vi "_Add A New Entry.vi"(4 "Tag Name":string="ChannelDescription", 5 "error in (no error)":errorcluster, 6 "Data":string, 7 "Parent Node":refnum<k20>, 8 "DOM document":refnum<k20>) -> (0 "error out":errorcluster, 2 "Parent Node out":refnum<k20>, 3 "DOM document out":refnum<k20>)   [LabVIEW 2015]
uses:
  <vilib>/xml/Close Reference(Node).vi
  <resource>/objmgr/DOMUserDefRef.rc
  <vilib>/xml/NI_XML.lvlib
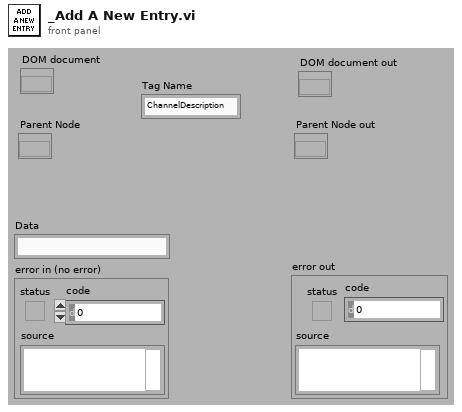
[diagram p1: front panel]
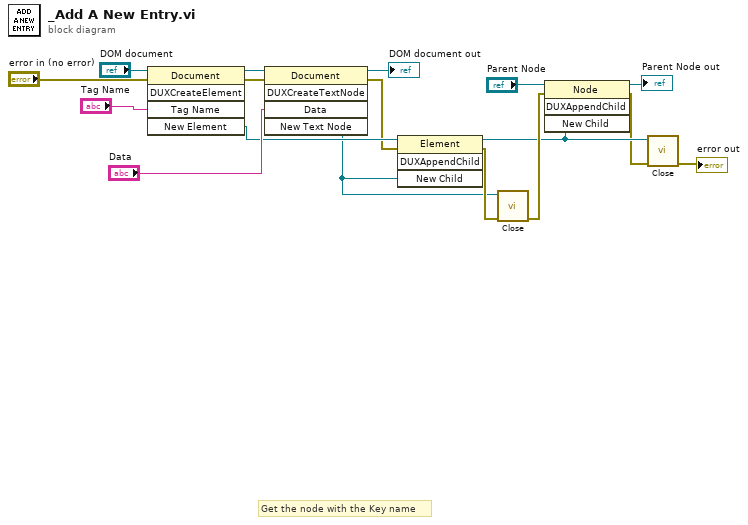
[diagram p0: block diagram]
diagram:
  # "Get the node with the Key name"
  n1 = invoke class="Document" method="DUXCreateElement"(reference="DOM document", error in="error in (no error)", "Tag Name"="Tag Name") -> (reference out=w15:refnum<k20>, error out=w14:errorcluster, "New Element"=w11:refnum<k20>)  [unwired: 2 in, 2 out]
  n2 = invoke class="Document" method="DUXCreateTextNode"(reference=w15, error in=w14, "Data"="Data") -> (reference out=→"DOM document out":refnum<k20>, error out=w10:errorcluster, "New Text Node"=w7:refnum<k20>)  [unwired: 2 in, 2 out]
  n3 = invoke class="Element" method="DUXAppendChild"(reference=w11, error in=w10, "New Child"=w7) -> (reference out=w5:refnum<k20>, error out=w8:errorcluster)  [unwired: 1 in, 2 out]
  n4 = call-poly <vilib>:"Close.vi"("error in (no error)"=w8, "node"=w7) -> ("error out"=w6:errorcluster)  [unwired: 7 in]
  n5 = invoke class="Node" method="DUXAppendChild"(reference="Parent Node", error in=w6, "New Child"=w5) -> (reference out=→"Parent Node out":refnum<k20>, error out=w4:errorcluster)  [unwired: 1 in, 2 out]
  n6 = call-poly <vilib>:"Close.vi"("error in (no error)"=w4, "node"=w5) -> ("error out"=→"error out":errorcluster)  [unwired: 7 in]
